vi "平行样集成干预数据组合(子VI).vi"(9 "污染物编码":string, 10 "数据输入":string[][](array[string]), 11 "小时数据发送次数":i32) -> (3 "输出组合":string)   [LabVIEW 2016, in "数据传输系统-02.lvlib"]
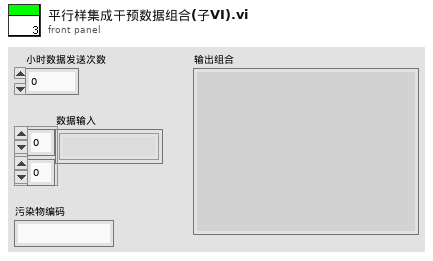
[diagram p1: front panel]
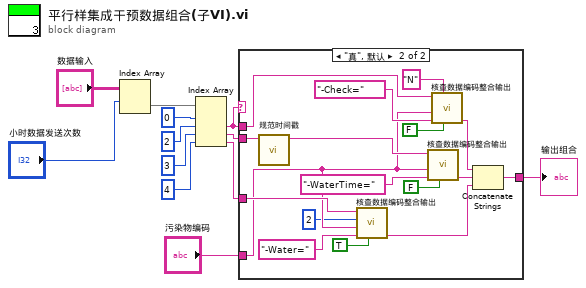
[diagram p0: block diagram]
diagram:
  n1 = Index Array(array="数据输入", index (row)="小时数据发送次数") -> (element=w5:string[])  [unwired: 1 in]
  n2 = Index Array(array=w5, index #1=0 ("索引"), index #2=2 ("索引"), index #3=3 ("索引"), index #4=4 ("索引")) -> (element #2=w2:string, element #3=w4:string, element #4=w3:string)  [unwired: 1 out]
  n3 = case shown="\"真\", 默认" w2 {
    selector: w2 -> [w13 _]
    tunnel: w2 -> [_ w29]
    tunnel: w3 -> [_ w23]
    tunnel: w4 -> [_ w21]
    tunnel: [w13 w16] -> w9
    tunnel: "污染物编码" -> [_ w15]
    frame "" {
    }
    frame "真", Default {
      n4 = call "规范时间戳.vi"("字符串"=w21) -> ("result string"=w20:string)  [unwired: 10 in]
      n5 = call "核查数据编码整合输出.vi"("字段结束"=TRUE, "数据类型"="-Water=", "污染物编码"=w15, "数据精度"=2, "数据值"=w23) -> ("编码输出"=w17:string)  [unwired: 6 in]
      n6 = call "核查数据编码整合输出.vi"("字段结束"=FALSE, "数据类型"="-WaterTime=", "污染物编码"=w15, "数据值"=w20) -> ("编码输出"=w18:string)  [unwired: 7 in]
      n7 = call "核查数据编码整合输出.vi"("字段结束"=FALSE, "数据标识"="N" ("字符串"), "数据类型"="-Check=", "污染物编码"=w15, "数据值"=w29) -> ("编码输出"=w19:string)  [unwired: 6 in]
      n8 = Concatenate Strings(w19, w18, w17) -> (w16:string)
    }
  }
  "输出组合" <- w9
